vi "Get Stream Frame Count.vi"(8 "error in (no error)":errorcluster, 11 "Camera in":refnum<class "Camera.lvclass">) -> (0 "error out":errorcluster, 2 "Frame Count (inc Errors)":u64, 3 "Camera":refnum<class "Camera.lvclass">)   [LabVIEW 2020, in "Camera.lvclass"]
doc: "Get the total number of frames that have been captured (including errors) since this streaming operation began."
uses:
  Camera.lvclass
  Camera.lvclass/Camera.ctl
  bin/gindustrialcam_32-1.dll
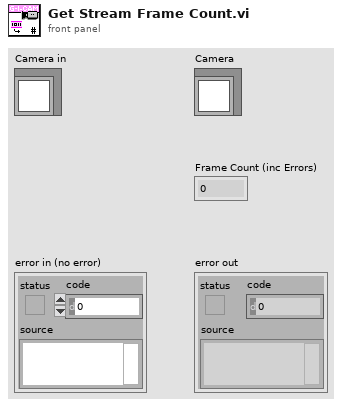
[diagram p1: front panel]
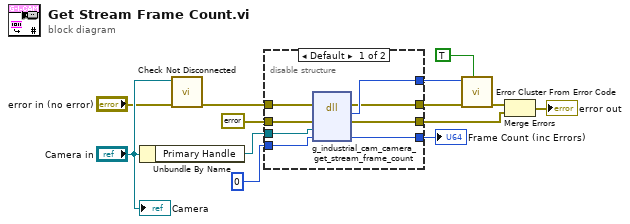
[diagram p0: block diagram]
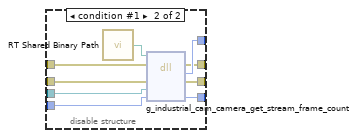
[diagram p2: hidden frame]
diagram:
  n1 = Unbundle By Name("Camera in") -> ("Primary Handle"=w9:refnum<data-value>)
  n2 = call "Check Not Disconnected.vi"("error in (no error)"="error in (no error)", "Camera in"="Camera in") -> ("error out"=w10:errorcluster)  [unwired: 9 in]
  n3 = disable-structure shown="Default" {
    disable-tunnel: w10 -> [w21 w30]
    disable-tunnel: w9 -> [w20 w29]
    disable-tunnel: errorcluster {"status"=FALSE, "code"=0, "source"=""} ("error constant") -> [w19 w28]
    disable-tunnel: [w18 w27] -> w6
    disable-tunnel: [w17 w26] -> w4
    disable-tunnel: [w16 w25] -> w3
    disable-tunnel: u64 0 ("count") -> [w15 w24]
    disable-tunnel: [w14 w23] -> w1
    frame condition #0 (active) {
      n4 = dll-call lib="C:/serenial/lib/g-industrial-camera/LabVIEW/g_industrial_cam/bin/gindustrialcam_*-1.*" fn="g_industrial_cam_camera_get_stream_frame_count"(error in=w21, "err"=w19, "edvr"=w20, "count"=w15) -> (error out=w16:errorcluster, "Mg_Error"=w17:i32, "err"=w18:errorcluster, "count"=w14:u64)  [unwired: 3 in, 1 out]
    }
    frame condition #1 {
      n5 = call "RT Shared Binary Path.vi"() -> ("Path"=w22:path)
      n6 = dll-call lib="C:/serenial/lib/g-industrial-camera/LabVIEW/g_industrial_cam/bin/gindustrialcam_*-1.*" fn="g_industrial_cam_camera_get_stream_frame_count"(path in=w22, error in=w30, "err"=w28, "edvr"=w29, "count"=w24) -> (error out=w25:errorcluster, "Mg_Error"=w26:i32, "err"=w27:errorcluster, "count"=w23:u64)  [unwired: 2 in, 1 out]
    }
  }
  "Frame Count (inc Errors)" <- w1
  n7 = call <vilib>:"Error Cluster From Error Code.vi"("show call chain? (False)"=TRUE, "error in (no error)"=w3, "error code (0)"=w4) -> ("error out"=w5:errorcluster)  [unwired: 6 in]
  n8 = Merge Errors(w5, w6) -> (→"error out":errorcluster)
  "Camera" <- "Camera in"
